vi "1D-Array_Mean_SD.vi"(7 "N":i32, 9 "Data Array":dbl[](array[numeric]), 11 "IN":dbl[][](array[numeric])) -> (3 "OUT":dbl[][](array[numeric]))   [LabVIEW 2018]
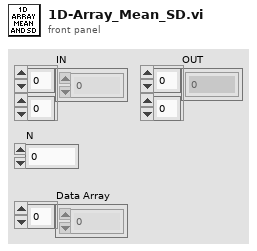
[diagram p1: front panel]
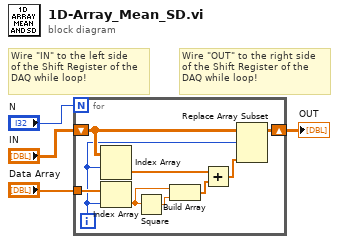
[diagram p0: block diagram]
diagram:
  # "Wire \"OUT\" to the right side\nof the Shift Register of the \nDAQ while loop!"
  # "Wire \"IN\" to the left side\nof the Shift Register of the\nDAQ while loop!"
  n1 = for {
    N: "N" -> [_]
    tunnel: "Data Array" -> [w13]
    shift-right: [w5] -> w3
    shift-left: "IN" -> [w12]
    i -> [w6]
    n2 = Index Array(array=w12, index (row)=w6) -> (element=w8:dbl[])  [unwired: 1 in]
    n3 = Index Array(array=w13, index=w6) -> (element=w10:dbl)
    n4 = Square(x=w10) -> (x^2=w11:dbl)
    n5 = Build Array(w10, w11) -> (w9:dbl[])
    n6 = Add(x=w8, y=w9) -> (x+y=w7:dbl[])
    n7 = Replace Array Subset(array=w12, new element=w7, index (row)=w6) -> (w5:dbl[][])  [unwired: 1 in]
  }
  "OUT" <- w3
